vi "CCD_Exposure 1-D.vi"(7 "CCD GPIB Address":u16=1, 8 "error in":errorcluster, 11 "CCD Parameters":T1={"Exposure Time (s)"=0.2, "Offset"=0.0, "BkgrdCrct"=FALSE, "Shutter"=FALSE, "Mode"=enum."Regular", "Repetition"=4, "dt or s"=0.0} {"dt or s" format="%#.6f"; "Repetition" min=1; "Offset" format="%#.2f"; "Exposure Time (s)" min=0.02 max=6000.0 format="%#.2f"}) -> (0 "Error Out":errorcluster, 1 "#PixelOverflow":u32, 2 "PixelOverflow":bool, 3 "The Data":dbl[](array[numeric])=[1198.0, 1190.0, 1193.0, 1194.0, 1189.0, 1188.0, 1196.0, 1190.0, 1202.0, 1191.0, 1193.0, 1192.0, 1199.0, 1189.0, 1194.0, 1189.0, 1197.0, 1191.0, 1187.0, 1192.0, 1195.0, 1189.0, 1195.0, 1191.0, 1199.0, 1194.0, 1192.0, 1191.0, 1193.0, 1197.0, 1193.0, 1193.0, 1194.0, 1200.0, 1191.0, 1190.0, 1187.0, 1195.0, 1189.0, 1188.0, 1191.0, 1194.0, 1187.0, 1192.0, 1198.0, 1193.0, 1190.0, 1192.0, 1190.0, 1193.0, 1191.0, 1190.0, 1191.0, 1189.0, 1192.0, 1194.0, 1190.0, 1193.0, 1193.0, 1191.0, 1194.0, 1182.0, 1190.0, 1188.0, 1199.0, 1192.0, 1196.0, 1195.0, 1186.0, 1189.0, 1188.0, 1185.0, 1194.0, 1187.0, 1193.0, 1194.0, 1190.0, 1189.0, 1189.0, 1187.0, 1196.0, 1195.0, 1191.0, 1197.0, 1192.0, 1200.0, 1187.0, 1194.0, 1189.0, 1193.0, 1195.0, 1196.0, 1186.0, 1192.0, 1190.0, 1194.0, 1194.0, 1190.0, 1191.0, 1193.0, 1197.0, 1197.0, 1185.0, 1199.0, 1190.0, 1195.0, 1196.0, 1184.0, 1193.0, 1193.0, 1193.0, 1191.0, 1189.0, 1190.0, 1199.0, 1193.0, 1191.0, 1194.0, 1191.0, 1192.0, 1186.0, 1190.0, 1194.0, 1189.0, 1194.0, 1190.0, 1191.0, 1192.0, 1192.0, 1196.0, 1192.0, 1192.0, 1189.0, 1193.0, 1198.0, 1186.0, 1191.0, 1193.0, 1187.0, 1194.0, 1190.0, 1190.0, 1191.0, 1189.0, 1194.0, 1195.0, 1189.0, 1192.0, 1185.0, 1193.0, 1192.0, 1192.0, 1189.0, 1191.0, 1191.0, 1190.0, 1196.0, 1194.0, 1193.0, 1191.0, 1189.0, 1191.0, 1196.0, 1192.0, 1192.0, 1189.0, 1196.0, 1191.0, 1193.0, 1192.0, 1188.0, 1190.0, 1194.0, 1192.0, 1185.0, 1191.0, 1194.0, 1191.0, 1189.0, 1195.0, 1192.0, 1196.0, 1190.0, 1193.0, 1191.0, 1189.0, 1194.0, 1195.0, 1191.0, 1187.0, 1190.0, 1196.0, 1196.0, 1192.0, 1197.0, 1191.0, 1189.0, 1192.0, 1192.0, 1200.0, 1192.0, 1193.0, 1190.0, 1192.0, 1187.0, 1198.0, 1186.0, 1196.0, 1201.0, 1199.0, 1200.0, 1191.0, 1196.0, 1200.0, 1192.0, 1191.0, 1193.0, 1185.0, 1192.0, 1194.0, 1186.0, 1190.0, 1188.0, 1189.0, 1201.0, 1197.0, 1191.0, 1194.0, 1193.0, 1194.0, 1195.0, 1198.0, 1200.0, 1192.0, 1192.0, 1193.0, 1193.0, 1195.0, 1187.0, 1193.0, 1192.0, 1187.0, 1189.0, 1186.0, 1191.0, 1197.0, 1191.0, 1200.0, 1194.0, 1192.0, 1187.0, 1196.0, 1191.0, 1191.0, 1196.0, 1187.0, 1190.0, 1193.0, 1189.0, 1193.0, 1190.0, 1188.0, 1188.0, 1190.0, 1197.0, 1188.0, 1191.0, 1195.0, 1188.0, 1191.0, 1188.0, 1194.0, 1193.0, 1187.0, 1200.0, 1192.0, 1197.0, 1190.0, 1196.0, 1200.0, 1191.0, 1189.0, 1193.0, 1189.0, 1186.0, 1196.0, 1185.0, 1198.0, 1195.0, 1186.0, 1191.0, 1197.0, 1191.0, 1193.0, 1195.0, 1193.0, 1191.0, 1198.0, 1189.0, 1183.0, 1200.0, 1197.0, 1192.0, 1192.0, 1192.0, 1196.0, 1191.0, 1190.0, 1194.0, 1188.0, 1198.0, 1193.0, 1195.0, 1190.0, 1187.0, 1192.0, 1191.0, 1195.0, 1188.0, 1190.0, 1191.0, 1187.0, 1189.0, 1185.0, 1189.0, 1196.0, 1198.0, 1191.0, 1190.0, 1196.0, 1197.0, 1193.0, 1187.0, 1186.0, 1195.0, 1191.0, 1193.0, 1192.0, 1196.0, 1190.0, 1192.0, 1192.0, 1192.0, 1190.0, 1195.0, 1192.0, 1191.0, 1193.0, 1197.0, 1184.0, 1190.0, 1188.0, 1192.0, 1194.0, 1190.0, 1193.0, 1195.0, 1195.0, 1194.0, 1189.0, 1193.0, 1191.0, 1194.0, 1186.0, 1189.0, 1192.0, 1191.0, 1182.0, 1190.0, 1197.0, 1194.0, 1188.0, 1193.0, 1191.0, 1186.0, 1194.0, 1197.0, 1193.0, 1191.0, 1187.0, 1194.0, 1194.0, 1191.0, 1189.0, 1195.0, 1194.0, 1189.0, 1196.0, 1187.0, 1186.0, 1192.0, 1194.0, 1196.0, 1191.0, 1193.0, 1191.0, 1188.0, 1190.0, 1199.0, 1198.0, 1196.0, 1196.0, 1190.0, 1194.0, 1191.0, 1194.0, 1187.0, 1195.0, 1190.0, 1194.0, 1196.0, 1194.0, 1189.0, 1193.0, 1189.0, 1194.0, 1189.0, 1195.0, 1192.0, 1194.0, 1193.0, 1191.0, 1197.0, 1187.0, 1189.0, 1189.0, 1188.0, 1197.0, 1192.0, 1189.0, 1193.0, 1194.0, 1183.0, 1202.0, 1187.0, 1192.0, 1184.0, 1188.0, 1186.0, 1193.0, 1189.0, 1195.0, 1189.0, 1193.0, 1197.0, 1189.0, 1194.0, 1191.0, 1194.0, 1192.0, 1191.0, 1191.0, 1196.0, 1194.0, 1190.0, 1193.0, 1192.0, 1195.0, 1197.0, 1198.0, 1193.0, 1202.0, 1196.0, 1194.0, 1194.0, 1190.0, 1193.0, 1190.0, 1195.0, 1192.0, 1187.0, 1194.0, 1197.0, 1190.0, 1194.0, 1189.0, 1198.0, 1192.0, 1191.0, 1192.0, 1192.0, 1191.0, 1191.0, 1193.0, 1191.0, 1191.0, 1198.0, 1186.0, 1192.0, 1185.0, 1185.0, 1188.0, 1194.0, 1196.0, 1194.0, 1195.0, 1190.0, 1194.0, 1191.0, 1190.0, 1195.0, 1191.0, 1191.0, 1195.0, 1192.0, 1194.0, 1201.0, 1187.0, 1191.0, 1195.0, 1187.0, 1192.0, 1192.0, 1193.0, 1200.0, 1188.0, 1189.0, 1189.0, 1197.0, 1189.0, 1188.0, 1197.0, 1195.0, 1191.0, 1189.0, 1190.0, 1195.0, 1189.0, 1191.0, 1194.0, 1186.0, 1192.0, 1190.0, 1191.0, 1188.0, 1195.0, 1192.0, 1191.0, 1191.0, 1199.0, 1190.0, 1190.0, 1190.0, 1192.0, 1187.0, 1193.0, 1197.0, 1197.0, 1186.0, 1193.0, 1189.0, 1192.0, 1197.0, 1184.0, 1187.0, 1188.0, 1192.0, 1192.0, 1192.0, 1189.0, 1192.0, 1190.0, 1194.0, 1191.0, 1186.0, 1196.0, 1194.0, 1189.0, 1193.0, 1191.0, 1186.0, 1189.0, 1193.0, 1195.0, 1196.0, 1197.0, 1199.0, 1194.0, 1190.0, 1193.0, 1194.0, 1190.0, 1198.0, 1196.0, 1194.0, 1195.0, 1194.0, 1184.0, 1188.0, 1195.0, 1197.0, 1190.0, 1194.0, 1190.0, 1191.0, 1195.0, 1198.0, 1188.0, 1193.0, 1194.0, 1195.0, 1198.0, 1195.0, 1191.0, 1197.0, 1192.0, 1198.0, 1190.0, 1196.0, 1191.0, 1194.0, 1188.0, 1189.0, 1198.0, 1192.0, 1198.0, 1195.0, 1185.0, 1191.0, 1193.0, 1192.0, 1197.0, 1195.0, 1195.0, 1195.0, 1193.0, 1190.0, 1190.0, 1190.0, 1198.0, 1195.0, 1191.0, 1194.0, 1190.0, 1190.0, 1194.0, 1194.0, 1195.0, 1192.0, 1190.0, 1194.0, 1195.0, 1192.0, 1192.0, 1194.0, 1189.0, 1192.0, 1193.0, 1188.0, 1194.0, 1195.0, 1196.0, 1193.0, 1192.0, 1201.0, 1191.0, 1198.0, 1197.0, 1191.0, 1192.0, 1191.0, 1194.0, 1193.0, 1188.0, 1192.0, 1189.0, 1183.0, 1189.0, 1190.0, 1192.0, 1189.0, 1196.0, 1193.0, 1197.0, 1185.0, 1193.0, 1189.0, 1191.0, 1196.0, 1195.0, 1193.0, 1193.0, 1191.0, 1189.0, 1193.0, 1192.0, 1192.0, 1192.0, 1190.0, 1191.0, 1193.0, 1193.0, 1197.0, 1195.0, 1189.0, 1193.0, 1188.0, 1194.0, 1197.0, 1194.0, 1195.0, 1196.0, 1190.0, 1194.0, 1188.0, 1197.0, 1195.0, 1191.0, 1195.0, 1192.0, 1194.0, 1188.0, 1190.0, 1197.0, 1197.0, 1191.0, 1187.0, 1197.0, 1191.0, 1193.0, 1188.0, 1191.0, 1194.0, 1193.0, 1195.0, 1192.0, 1195.0, 1189.0, 1193.0, 1193.0, 1195.0, 1190.0, 1192.0, 1196.0, 1188.0, 1187.0, 1193.0, 1192.0, 1192.0, 1194.0, 1185.0, 1199.0, 1190.0, 1193.0, 1191.0, 1198.0, 1189.0, 1190.0, 1191.0, 1190.0, 1193.0, 1195.0, 1186.0, 1190.0, 1193.0, 1191.0, 1189.0, 1197.0, 1193.0, 1198.0, 1190.0, 1192.0, 1193.0, 1191.0, 1196.0, 1193.0, 1196.0, 1190.0, 1190.0, 1198.0, 1192.0, 1199.0, 1198.0, 1190.0, 1191.0, 1191.0, 1196.0, 1190.0, 1196.0, 1195.0, 1191.0, 1196.0, 1195.0, 1193.0, 1190.0, 1190.0, 1195.0, 1193.0, 1187.0, 1197.0, 1185.0, 1191.0, 1189.0, 1191.0, 1193.0, 1192.0, 1188.0, 1196.0, 1193.0, 1191.0, 1193.0, 1193.0, 1190.0, 1192.0, 1192.0, 1192.0, 1195.0, 1191.0, 1195.0, 1189.0, 1189.0, 1191.0, 1191.0, 1185.0, 1192.0, 1191.0, 1193.0, 1201.0, 1199.0, 1197.0, 1206.0, 1201.0, 1207.0, 1200.0, 1198.0, 1195.0, 1188.0, 1194.0, 1186.0, 1190.0, 1197.0, 1188.0, 1193.0, 1196.0, 1193.0, 1192.0, 1192.0, 1188.0, 1196.0, 1186.0, 1193.0, 1194.0, 1188.0, 1190.0, 1190.0, 1192.0, 1190.0, 1191.0, 1191.0, 1200.0, 1192.0, 1199.0, 1193.0, 1190.0, 1190.0, 1199.0, 1187.0, 1193.0, 1190.0, 1188.0, 1194.0, 1194.0, 1196.0, 1194.0, 1195.0, 1190.0, 1187.0, 1187.0, 1196.0, 1193.0, 1199.0, 1190.0, 1193.0, 1193.0, 1191.0, 1198.0, 1192.0, 1193.0, 1192.0, 1193.0, 1189.0, 1189.0, 1197.0, 1189.0, 1194.0, 1193.0, 1192.0, 1185.0, 1198.0, 1193.0, 1189.0, 1192.0, 1193.0, 1196.0, 1190.0, 1195.0, 1189.0, 1196.0, 1198.0, 1190.0, 1191.0, 1193.0, 1186.0, 1189.0, 1195.0, 1188.0, 1197.0, 1188.0, 1191.0, 1185.0, 1190.0, 1193.0, 1188.0, 1198.0, 1192.0, 1193.0, 1194.0, 1194.0, 1189.0, 1184.0, 1193.0, 1199.0, 1193.0, 1192.0, 1193.0, 1190.0, 1196.0, 1191.0, 1192.0, 1189.0, 1194.0, 1188.0, 1189.0, 1190.0, 1190.0, 1192.0, 1195.0, 1188.0, 1190.0, 1192.0, 1189.0, 1197.0, 1192.0, 1194.0, 1187.0, 1196.0, 1192.0, 1194.0, 1185.0, 1187.0, 1187.0, 1191.0, 1195.0, 1190.0, 1186.0, 1183.0, 1194.0, 1194.0, 1192.0, 1192.0, 1188.0, 1193.0, 1195.0, 1189.0, 1190.0, 1191.0, 1192.0, 1196.0, 1186.0, 1195.0, 1191.0, 1185.0, 1191.0, 1187.0, 1190.0, 1188.0, 1189.0, 1187.0, 1196.0, 1191.0, 1190.0, 1191.0, 1190.0, 1196.0, 1195.0, 1186.0, 1187.0, 1187.0, 1188.0, 1194.0, 1192.0, 1192.0, 1192.0, 1189.0, 1192.0, 1191.0, 1188.0, 1188.0, 1187.0, 1187.0, 1190.0, 1186.0, 1191.0, 1195.0, 1192.0, 1196.0, 1193.0, 1192.0, 1191.0, 1189.0, 1187.0, 1193.0, 1188.0, 1189.0, 1194.0, 1191.0, 1185.0, 1193.0, 1191.0, 1196.0, 1196.0, 1199.0, 1195.0, 1211.0] format="%.2f", 4 "GPIB Status":i16=-1, 5 "Exposuretime (s) out":dbl format="%.2f", 6 "Setup String":string="ldu,0,256,16;sdu,0,1024,1024;cl0;omrm;sron")   [LabVIEW 2020]
uses:
  Globals and TypeDefs/Type Definitions.llb/CCDParameter.ctt
  Globals and TypeDefs/gDetector.vi
panel:
  out "Shot #":i32
  out "Repetition":u8=4 min=4
  out "Array Length":i32=1024
  out "Plot":i32[][](graph)
  # "of"
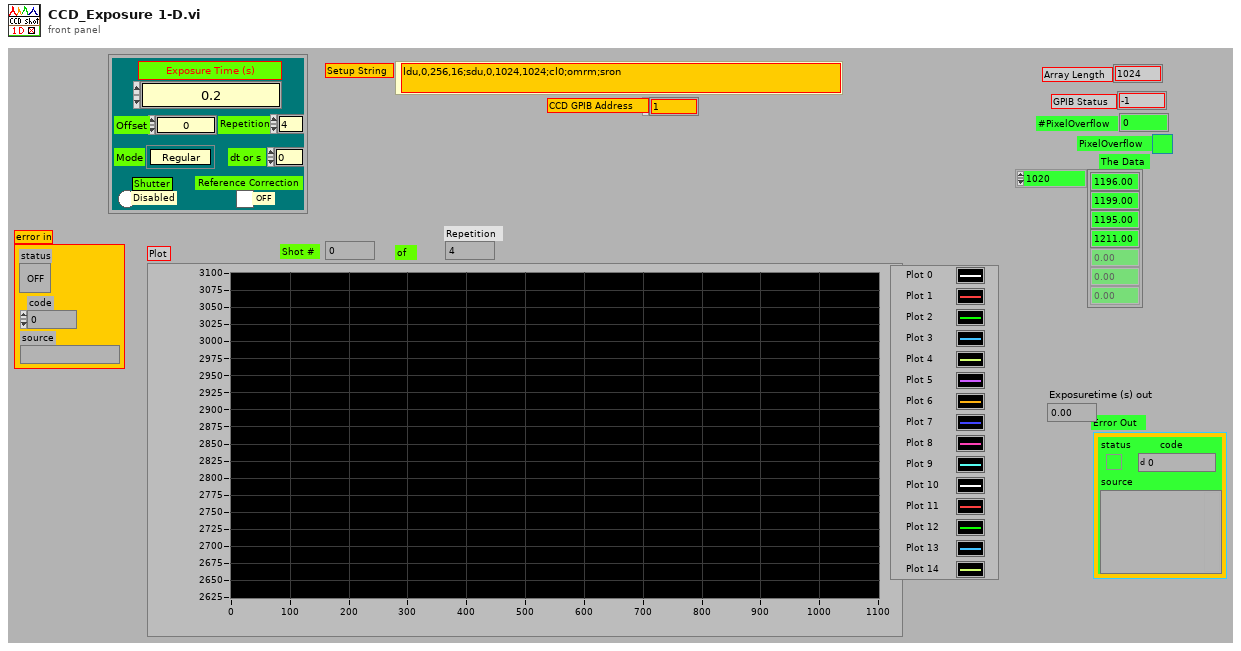
[diagram p1: front panel]
types:
  T1 = typedef "CCDParameter.ctt" = cluster{"Exposure Time (s)":dbl, "Offset":dbl, "BkgrdCrct":bool, "Shutter":bool, "Mode":enum8{"Regular", "OverExp Cor", "SpikeRemove", "ForCalibration"}, "Repetition":u16, "dt or s":dbl}
  T2 = enum8{"Regular", "OverExp Cor", "SpikeRemove", "ForCalibration"}
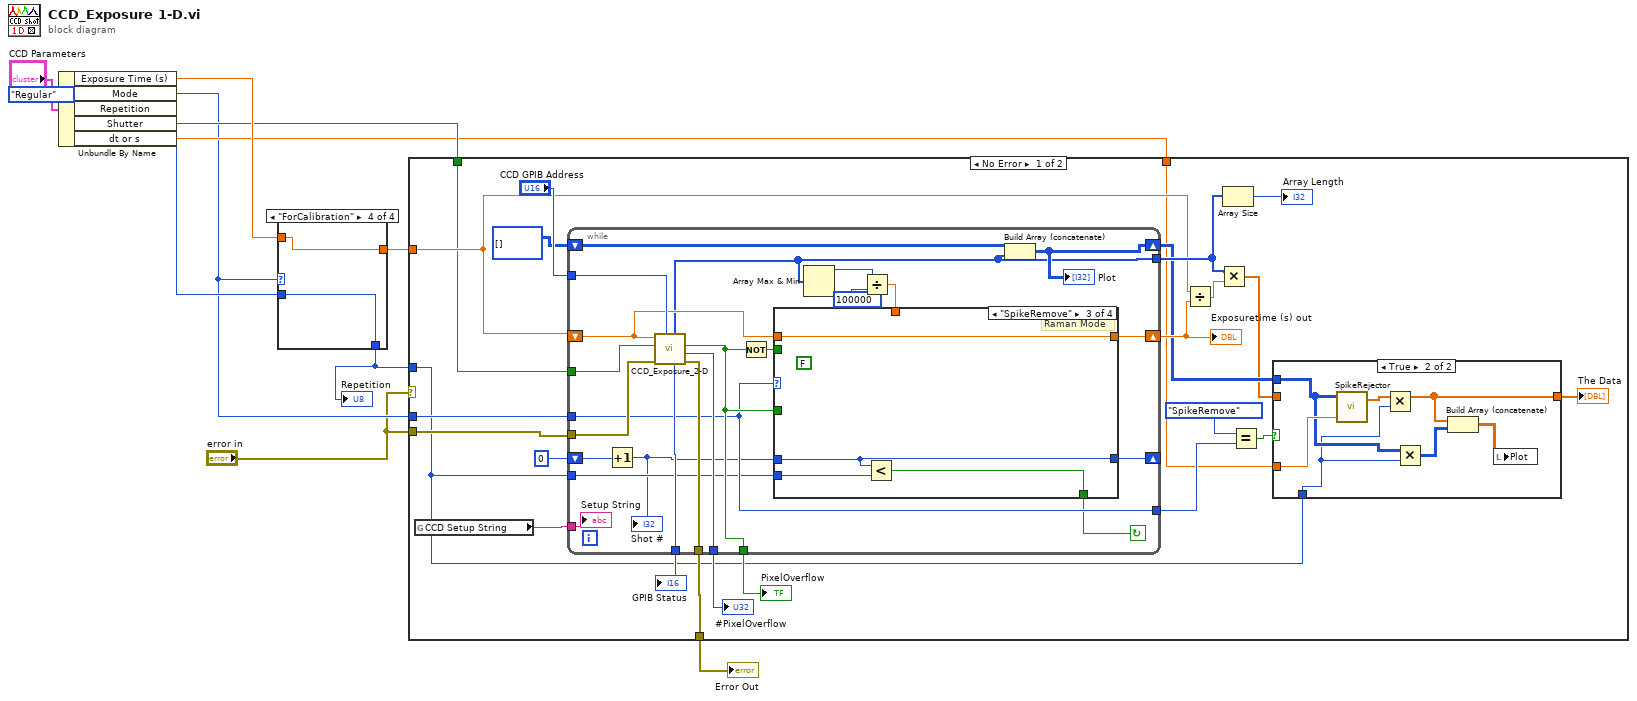
[diagram p0: block diagram]
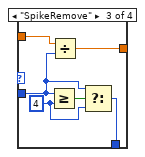
[diagram p4: hidden frame]
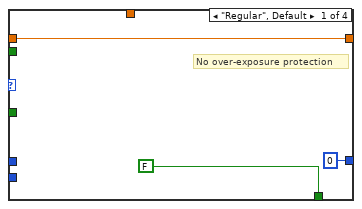
[diagram p6: hidden frame]
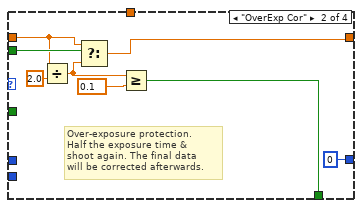
[diagram p7: hidden frame]
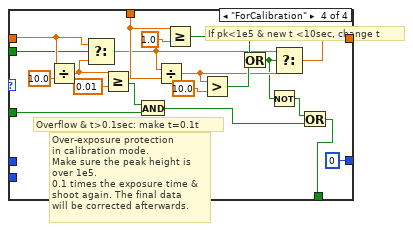
[diagram p8: hidden frame]
diagram:
  (unwired) T2."Regular" ("Mode")
  n1 = Unbundle By Name("CCD Parameters") -> ("Exposure Time (s)"=w7:dbl, "Mode"=w2:T2, "Repetition"=w4:u16, "Shutter"=w6:bool, "dt or s"=w5:dbl)
  n2 = case shown="\"ForCalibration\"" w2 {
    tunnel: w7 -> [w12 w14 w20 w22]
    tunnel: w4 -> [w11 w13 w17 w21]
    tunnel: [w12 w14 w19 w22] -> w9
    tunnel: [w11 w13 w15 w21] -> w3
    frame "Regular", Default {
    }
    frame "OverExp Cor" {
    }
    frame "SpikeRemove" {
      w16 = u8 4 ("y")
      n3 = Greater Or Equal?(x=w17, y=w16) -> (x >= y?=w18:bool)
      n4 = Divide(x=w20, y=w17) -> (x/y=w19:dbl)
      n5 = Select(t=w17, s=w18, f=w16) -> (s? t:f=w15:u16)
    }
    frame "ForCalibration" {
    }
  }
  "Repetition" <- w3
  n6 = case shown="No Error" "error in" {
    tunnel: "error in" -> [w38 w113]
    tunnel: [w37 w113] -> w10
    tunnel: w2 -> [w29 _]
    tunnel: w3 -> [w27 _]
    tunnel: w9 -> [w28 _]
    tunnel: w6 -> [w26 _]
    tunnel: w5 -> [w25 _]
    frame No Error {
      n7 = global read "gDetector.vi" "CCD Setup String"() -> (w24:string)
      n8 = while {
        tunnel: w24 -> [w65]
        tunnel: [w56] -> w39
        tunnel: [w63] -> w43
        tunnel: [w66] -> w44
        tunnel: [w67] -> w37
        tunnel: [w68] -> w45
        tunnel: "CCD GPIB Address" -> [w75]
        shift-left: w28 -> [w74]
        shift-right: [w69] -> w42
        tunnel: w38 -> [w76]
        tunnel: w26 -> [w77]
        shift-right: [w64] -> _
        shift-left: 0 -> [w58]
        shift-right: [w61] -> w32
        shift-left: i32[][] [] -> [w62]
        tunnel: [w60] -> w34
        tunnel: w29 -> [w60]
        tunnel: w27 -> [w59]
        stop <- w55 continue-if-true
        n9 = Increment(x=w58) -> (x+1=w57:i32)
        "Shot #" <- w57
        n10 = call "CCD_Exposure_2-D.vi"("CCD GPIB Address"=w75, "error in"=w76, "Shutter Enabled"=w77, "Exposuretime (s)"=w74) -> ("Error Out"=w67:errorcluster, "#PixelOverflow"=w66:u32, "PixelOverflow"=w63:bool, "SD"=w68:i32, "1-D data"=w56:i32[])  [unwired: 1 in, 2 out]
        n11 = Not(x=w63) -> (.not. x?=w73:bool)
        n12 = Array Max & Min(array=w56) -> (max value=w72:i32)  [unwired: 3 out]
        n13 = Divide(x=w72, y=100000) -> (x/y=w70:dbl)
        n14 = case shown="\"SpikeRemove\"" w60 {
          tunnel: [w80 w82 w92 w100] -> w69
          tunnel: w74 -> [w80 w84 w92 w109]
          tunnel: [FALSE w86 w91 w98] -> w55
          tunnel: w73 -> [_ w85 _ w108]
          tunnel: w70 -> [_ _ _ w106]
          tunnel: [0 0 w89 0] -> w64
          tunnel: w63 -> [_ _ _ w96]
          tunnel: w59 -> [_ _ w90 _]
          tunnel: w57 -> [_ _ w89 _]
          frame "Regular", Default {
            # "No over-exposure protection"
          }
          frame "OverExp Cor" {
            # "Over-exposure protection.\nHalf the exposure time &\nshoot again. The final data\nwill be corrected afterwards."
            n15 = Divide(x=w84, y=2.0) -> (x/y=w83:dbl)
            n16 = Select(t=w84, s=w85, f=w83) -> (s? t:f=w82:dbl)
            n17 = Greater Or Equal?(x=w83, y=0.1) -> (x >= y?=w86:bool)
          }
          frame "SpikeRemove" {
            (unwired) FALSE
            # "Raman Mode"
            n18 = Less?(x=w89, y=w90) -> (x < y?=w91:bool)
          }
          frame "ForCalibration" {
            # "If pk<1e5 & new t <10sec, change t"
            # "Overflow & t>0.1sec: make t=0.1t"
            # "Over-exposure protection\nin calibration mode. \nMake sure the peak height is \nover 1e5.\n0.1 times the exposure time &\nshoot again. The final data\nwill be corrected afterwards."
            n19 = Divide(x=w109, y=10.0) -> (x/y=w110:dbl)
            n20 = Select(t=w109, s=w108, f=w110) -> (s? t:f=w102:dbl)
            n21 = Greater Or Equal?(x=w110, y=0.01) -> (x >= y?=w97:bool)
            n22 = And(x=w97, y=w96) -> (x .and. y?=w95:bool)
            n23 = Divide(x=w102, y=w106) -> (x/y=w101:dbl)
            n24 = Greater Or Equal?(x=w106, y=1.0) -> (x >= y?=w103:bool)
            n25 = Greater?(x=w101, y=10.0) -> (0:w104:bool)
            n26 = Or(x=w103, y=w104) -> (x .or. y?=w93:bool)
            n27 = Not(x=w93) -> (.not. x?=w94:bool)
            n28 = Select(t=w102, s=w93, f=w101) -> (s? t:f=w100:dbl)
            n29 = Or(x=w94, y=w95) -> (x .or. y?=w98:bool)
          }
        }
        n30 = Build Array (concatenate)(w62, w56) -> (w61:i32[][])
        "Plot" <- w61
        "Setup String" <- w65
      }
      "PixelOverflow" <- w43
      "#PixelOverflow" <- w44
      "GPIB Status" <- w45
      "Exposuretime (s) out" <- w42
      n31 = Divide(x=w28, y=w42) -> (x/y=w41:dbl)
      n32 = Multiply(x=w39, y=w41) -> (x*y=w31:dbl[])
      n33 = Array Size(array=w39) -> (size(s)=→"Array Length":i32)
      n34 = Equal?(x=T2."SpikeRemove" ("Mode"), y=w34) -> (x = y?=w33:bool)
      n35 = case shown="True" w33 {
        tunnel: w25 -> [_ w54]
        tunnel: w32 -> [_ w50]
        tunnel: w31 -> [w47 _]
        tunnel: [w47 w52] -> w30
        tunnel: w27 -> [_ w49]
        frame False {
        }
        frame True {
          n36 = call "SpikeRejector.vi"("SigmaFactor"=w54, "Input Array"=w50) -> ("Final Array"=w53:dbl[])  [unwired: 2 in, 1 out]
          n37 = Multiply(x=w53, y=w49) -> (x*y=w52:dbl[])
          n38 = Multiply(x=w50, y=w49) -> (x*y=w48:i32[][])
          n39 = Build Array (concatenate)(w52, w48) -> (w51:dbl[][])
          n40 = local write "Plot"(w51) -> ()
        }
      }
      "The Data" <- w30
    }
    frame Error {
    }
  }
  "Error Out" <- w10
